vi "Quality_Traceability.vi"() -> ()   [LabVIEW 2020]
doc: "Fonction :\n\nCe modèle peut être intégré très facilement à un subpannel à l'aide des fonctions de la palette Code Template >> Dynamic VI and Subpanel de la VIBOX"
uses:
  System.Windows.Forms
  <vilib>/Utility/NIReport.llb/Report Type.ctl
  <vilib>/Utility/NIReport.llb/Append Text Table to Report (wrap).vi
  <vilib>/DataGrid for LabVIEW/source/DataTable/DataTable.lvclass
  <vilib>/DataGrid for LabVIEW/source/DataGridView/DataGridView.lvclass
  C:/Program Files (x86)/National Instruments/LabVIEW 2020/examples/DataGrid for LabVIEW/DataGrid.lvlib
  <vilib>/DataGrid for LabVIEW/source/Events/CellClick/CellClick.lvclass
  <vilib>/Utility/NIReport.llb/NI_report.lvclass
  <vilib>/Utility/NIReport.llb/NI_ReportGenerationCore.lvlib
panel:
  out "data":string[][](array[string])
  in  "截至日期":timestamp format="%<%x>T"
  in  "起始日期":timestamp caption="日期范围" format="%<%x>T"
  out "Stop":bool
  out "row":i32
  in  "加工状态":u16(ring) caption="Enum 3" items=["", "OK", "NG"]
  in  "生产编号":string
  in  "操作员":string
  in  "产品型号":u16(ring) caption="Enum 3" items=["", "R128", "R527", "R538", "R544", "R563X", "R92A"]
  in  "设备名称":u16(ring) caption="Enum 3" items=["", "芯轴分总成磨合台", "上管柱组件装配", "上管柱上转向轴合成", "滑移力检测", "芯轴分总成NVH", "上转向轴组件装配", "上下管柱总成装配", "滑移力复检", "最终性能试验台", "传感器对中台", "电机装配", "中间轴装配", "GP12（340）", "ECU装配", "激光打标机"]
  in  "追溯码":string
  in  "详细信息":bool
  in  "搜索按钮":bool
  out "Stop<user event>":refnum<user-event>
  in  "质量追溯":refnum<k24>(container)
  in  "导出全部行":bool
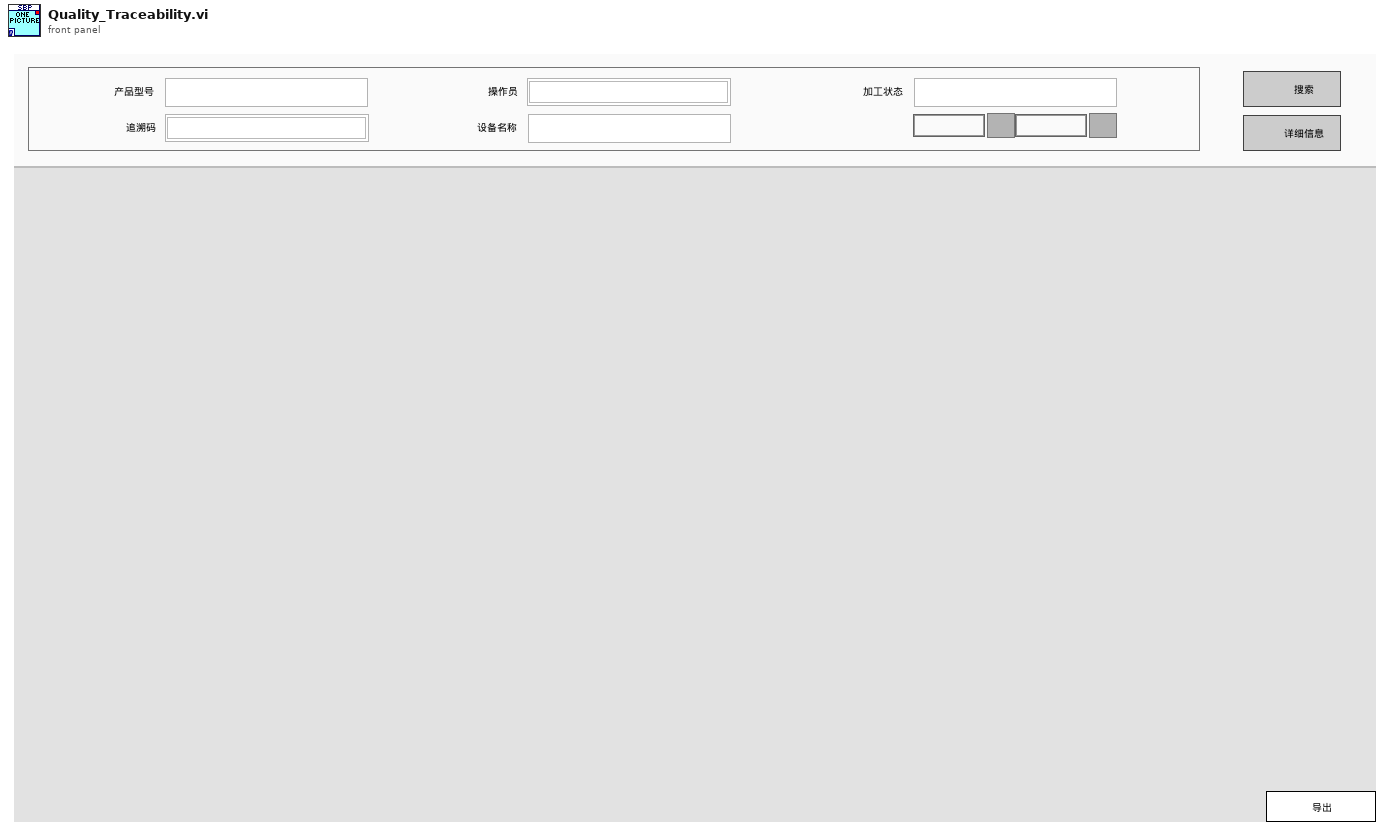
[diagram p1: front panel]
types:
  T1 = typedef "NI_ReportGenerationCore.lvlib/Report Type.ctl" = enum16{"HTML", "Word", "Excel"}
  T2 = enum16{"maximized", "minimized", "normal", "no change"}
  T3 = typedef "DataGrid.lvlib/GridColumn.lvclass/ColumnDefinition.ctl" = cluster{"name":string, "caption":string, "datatype":T4, "Params":string, "AutoSizeMode":i32, "FillWeight":sgl, "MinWidth":u32, "tooltip":string}
  T4 = typedef "DataGrid.lvlib/GridColumn.lvclass/ColumnType.ctl" = enum16{"string", "image", "check", "numeric", "timestamp", "button", "combo", "link"}
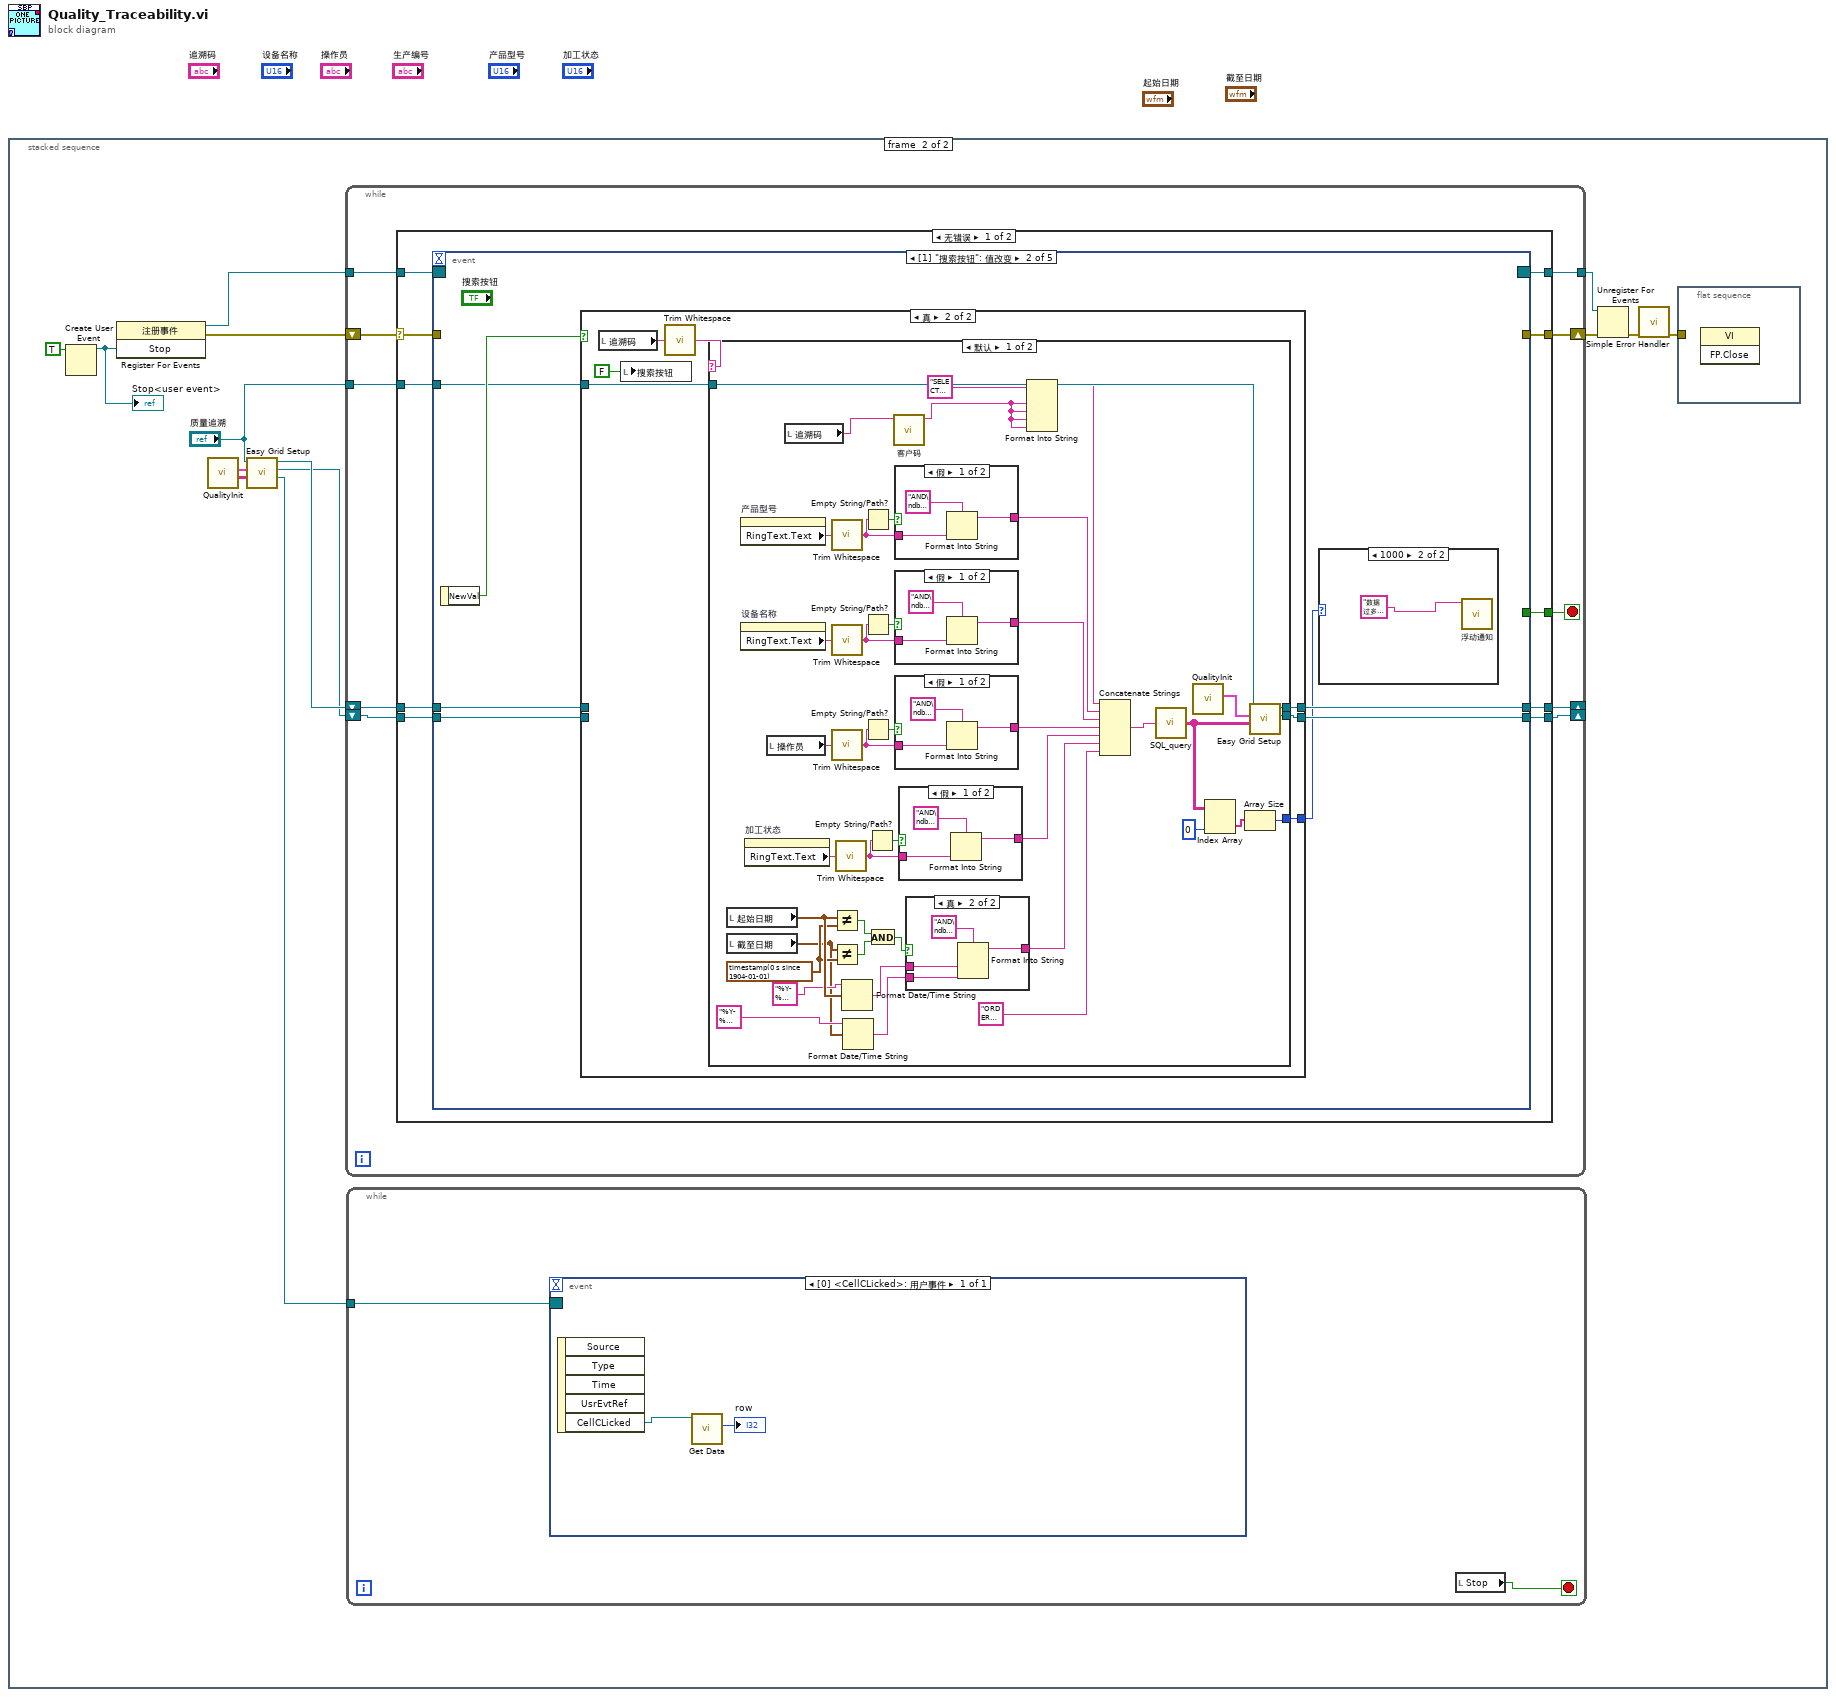
[diagram p0: block diagram]
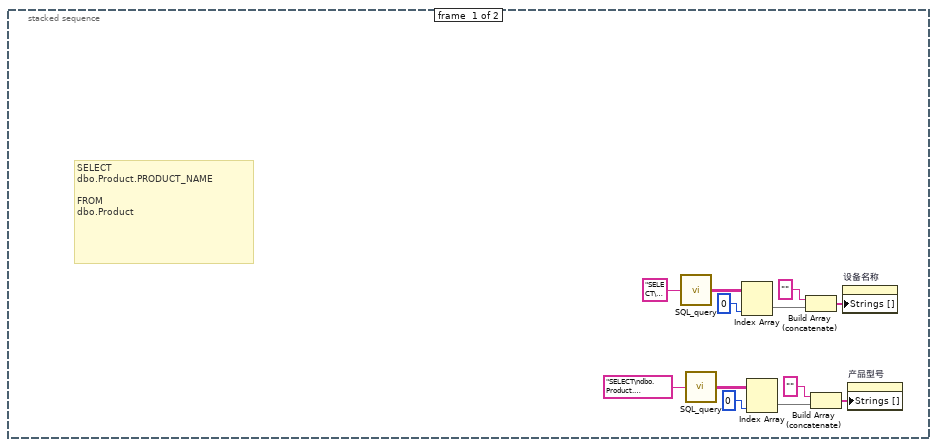
[diagram p2: hidden frame]
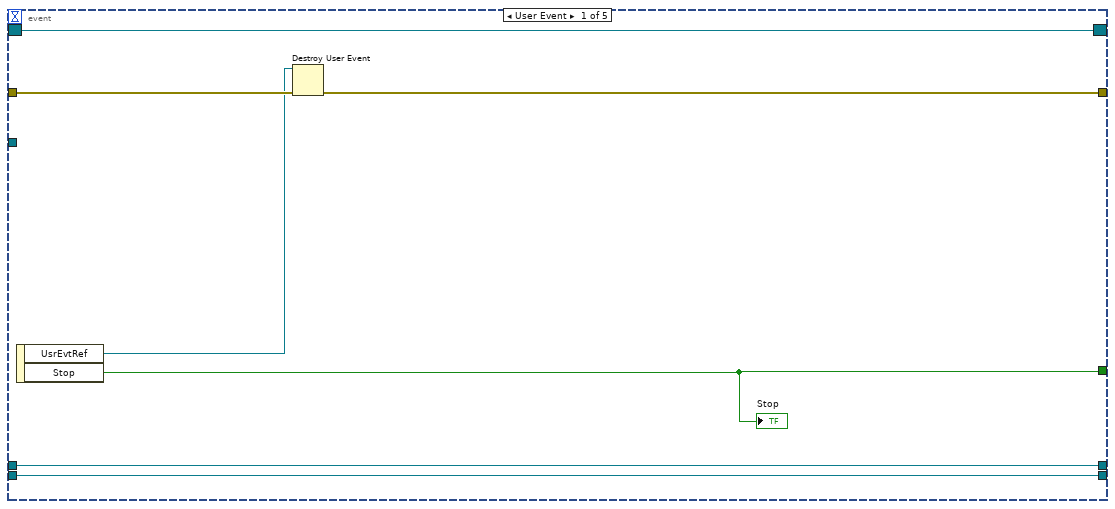
[diagram p3: hidden frame]
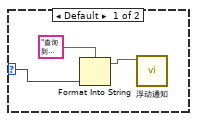
[diagram p4: hidden frame]
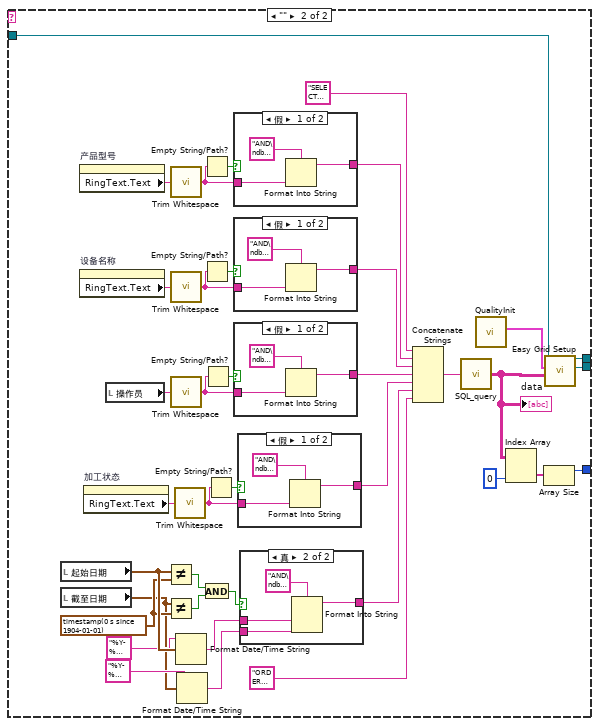
[diagram p11: hidden frame]
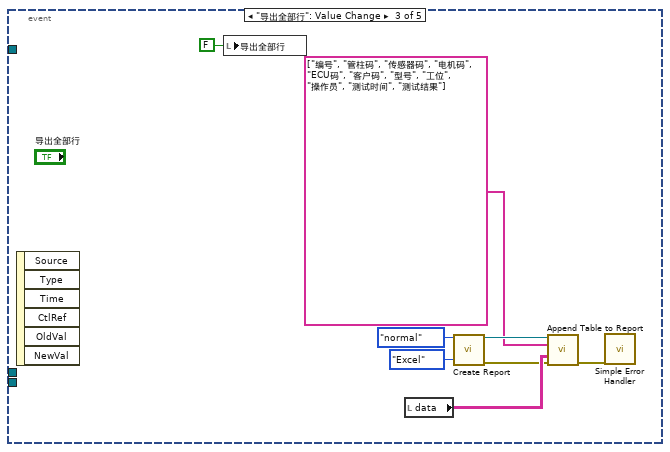
[diagram p17: hidden frame]
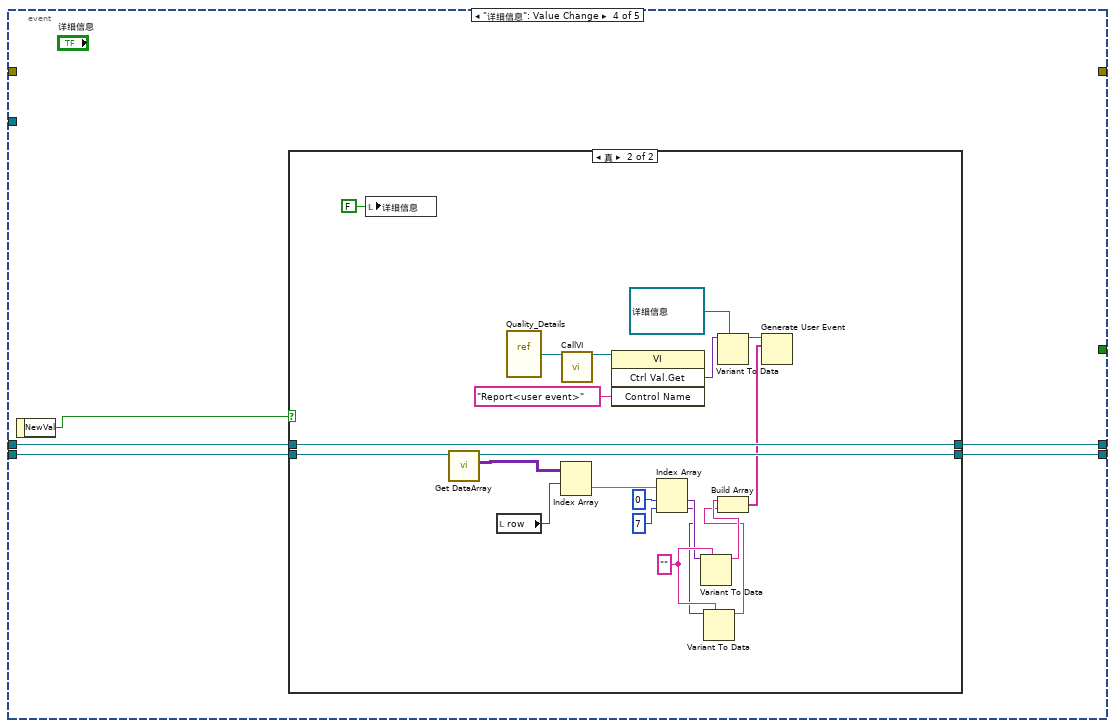
[diagram p18: hidden frame]
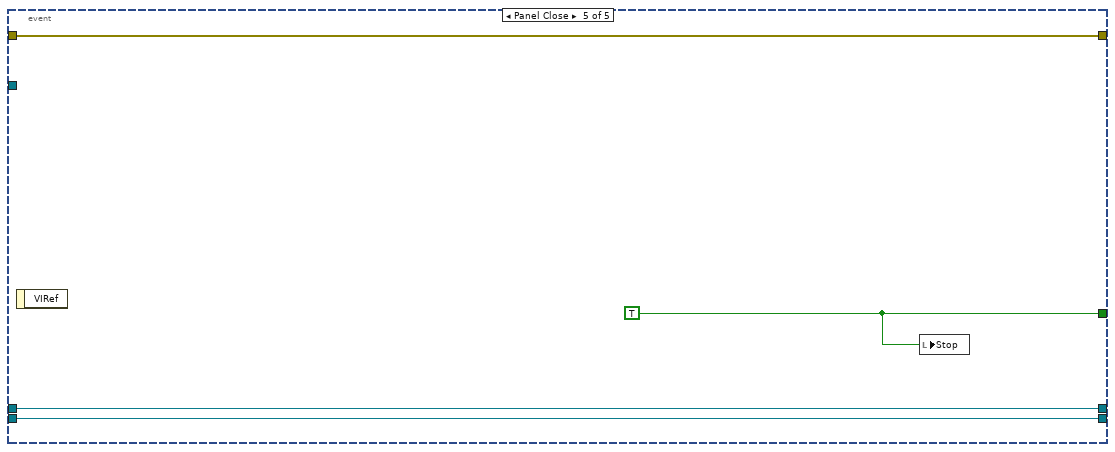
[diagram p20: hidden frame]
diagram:
  n1 = stacked-sequence {
    frame #0 {
      # "SELECT\ndbo.Product.PRODUCT_NAME\n\nFROM\ndbo.Product"
      n2 = call "SQL_query.vi"("SQL query"="SELECT\ndbo.Device.DEVICE_NAME\n\nFROM\ndbo.Device\n") -> ("data"=w11:string[][])  [unwired: 3 in, 1 out]
      n3 = call "SQL_query.vi"("SQL query"="SELECT\ndbo.Product.PRODUCT_NAME\n\nFROM\ndbo.Product\n") -> ("data"=w3:string[][])  [unwired: 3 in, 1 out]
      n4 = Index Array(array=w11, index (col)=0 ("禁用的索引 (列)")) -> (element=w10:string[])  [unwired: 1 in]
      n5 = Index Array(array=w3, index (col)=0 ("禁用的索引 (列)")) -> (element=w4:string[])  [unwired: 1 in]
      n6 = Build Array (concatenate)("", w10) -> (w8:string[])
      n7 = Build Array (concatenate)("", w4) -> (w1:string[])
      n8 = property on="设备名称" class="Ring (严格)"("Strings []"=w8) -> ()  [unwired: 2 in, 2 out]
      n9 = property on="产品型号" class="Ring (严格)"("Strings []"=w1) -> ()  [unwired: 2 in, 2 out]
    }
    frame #1 {
      n10 = Create User Event(user event datatype=TRUE ("Stop")) -> (user event=w24:refnum<user-event>)  [unwired: 1 in, 1 out]
      "Stop<user event>" <- w24
      n11 = register-events(w24) -> (reference out=w23:refnum<event-registration>, error out=w19:errorcluster)  [unwired: 2 in]
      n12 = call "QualityInit.vi"() -> ("DataSource Data"=w17:string[][], "ColumnSetup"=w18:T3[])  [unwired: 10 in]
      n13 = call <vilib>:"Easy Grid Setup.vi"("DataSource Data"=w17, "ColumnSetup"=w18, "DataGridView"="质量追溯") -> ("registeredEvents"=w15:refnum<event-registration>, "DataTable out"=w13:refnum<class "DataTable.lvclass">, "DataGrid out"=w14:refnum<class "DataGridView.lvclass">)  [unwired: 5 in, 1 out]
      n14 = while {
        tunnel: w23 -> [w37]
        tunnel: [w36] -> w26
        shift-right: [w39] -> w22
        shift-left: w19 -> [w40]
        tunnel: "质量追溯" -> [w35]
        shift-right: [w34] -> _
        shift-left: w14 -> [w32]
        shift-right: [w33] -> _
        shift-left: w13 -> [w31]
        stop <- w38 stop-if-true
        n15 = case shown="无错误" w40 {
          selector: w40 -> [w47 w232]
          tunnel: [w46 w232] -> w39
          tunnel: [w48 TRUE] -> w38
          tunnel: w37 -> [w49 w231]
          tunnel: [w50 w231] -> w36
          tunnel: w35 -> [w45 _]
          tunnel: [w44 w230] -> w34
          tunnel: [w43 w229] -> w33
          tunnel: w32 -> [w42 w230]
          tunnel: w31 -> [w41 w229]
          frame No Error {
            n16 = event shown="[1] \"搜索按钮\": 值改变" {
              selector: w49 -> [w57 _ _ _ _]
              dyn-events: [w57 _ _ _ _] -> w50
              timeout: _ -> [_ _ _ _ _]
              tunnel: [w54 _ _ _ w227] -> w48
              tunnel: w47 -> [w56 _ _ _ w228]
              tunnel: [w53 _ _ _ w228] -> w46
              tunnel: w45 -> [_ w63 _ _ _]
              tunnel: [w52 w62 _ w199 w226] -> w44
              tunnel: [w51 w61 _ w197 w225] -> w43
              tunnel: w42 -> [w52 w60 _ w200 w226]
              tunnel: w41 -> [w51 w59 _ w198 w225]
              event User Event {
                n17 = event-data() -> ("UsrEvtRef"=w55:refnum<user-event>, "Stop"=w54:bool)  [unwired: 1 out]
                "Stop" <- w54
                n18 = Destroy User Event(user event=w55, error in=w56) -> (error out=w53:errorcluster)
              }
              event "搜索按钮": Value Change {
                n19 = event-data() -> ("NewVal"=w64:bool)  [unwired: 1 out]
                n20 = case shown="真" w64 {
                  tunnel: w63 -> [_ w76]
                  tunnel: [w70 w73] -> w62
                  tunnel: [w69 w72] -> w61
                  tunnel: w60 -> [w70 _]
                  tunnel: w59 -> [w69 _]
                  tunnel: [_ w71] -> w58
                  frame False {
                  }
                  frame True {
                    n21 = local read "追溯码"() -> (w75:string)
                    n22 = local write "搜索按钮"(FALSE ("确定按钮")) -> ()
                    n23 = call <vilib>:"Trim Whitespace.vi"("string"=w75) -> ("trimmed string"=w74:string)  [unwired: 1 in]
                    n24 = case shown="默认" w74 {
                      tunnel: w76 -> [w108 w172]
                      tunnel: [w99 w170] -> w73
                      tunnel: [w98 w169] -> w72
                      tunnel: [w81 w136] -> w71
                      frame Default {
                        w87 = timestamp(0 s since 1904-01-01) ("起始日期")
                        n25 = local read "起始日期"() -> (w90:timestamp)
                        n26 = local read "截至日期"() -> (w82:timestamp)
                        n27 = property on="产品型号" class="Ring (严格)"() -> ("RingText.Text"=w118:string)  [unwired: 2 in, 2 out]
                        n28 = property on="设备名称" class="Ring (严格)"() -> ("RingText.Text"=w117:string)  [unwired: 2 in, 2 out]
                        n29 = property on="加工状态" class="Ring (严格)"() -> ("RingText.Text"=w102:string)  [unwired: 2 in, 2 out]
                        n30 = local read "操作员"() -> (w116:string)
                        n31 = local read "追溯码"() -> (w96:string)
                        n32 = call <vilib>:"Trim Whitespace.vi"("string"=w118) -> ("trimmed string"=w106:string)  [unwired: 1 in]
                        n33 = call <vilib>:"Trim Whitespace.vi"("string"=w117) -> ("trimmed string"=w105:string)  [unwired: 1 in]
                        n34 = call <vilib>:"Trim Whitespace.vi"("string"=w116) -> ("trimmed string"=w104:string)  [unwired: 1 in]
                        n35 = Not Equal?(x=w90, y=w87) -> (x != y?=w92:bool)
                        n36 = Not Equal?(x=w82, y=w87) -> (x != y?=w93:bool)
                        n37 = call <vilib>:"Trim Whitespace.vi"("string"=w102) -> ("trimmed string"=w101:string)  [unwired: 1 in]
                        n38 = Format Date/Time String(time format string (%c)="%Y-%m-%d 00:00:00.000" ("时间格式字符串(%c)"), seconds (now)=w90) -> (date/time string=w89:string)  [unwired: 1 in]
                        n39 = Format Date/Time String(time format string (%c)="%Y-%m-%d 23:59:59.999" ("时间格式字符串(%c)"), seconds (now)=w82) -> (date/time string=w88:string)  [unwired: 1 in]
                        n40 = Empty String/Path?(string/path=w106) -> (empty?=w113:bool)
                        n41 = Empty String/Path?(string/path=w105) -> (empty?=w114:bool)
                        n42 = Empty String/Path?(string/path=w104) -> (empty?=w115:bool)
                        n43 = Empty String/Path?(string/path=w101) -> (empty?=w103:bool)
                        n44 = And(x=w92, y=w93) -> (x .and. y?=w91:bool)
                        n45 = call "客户码.vi"("追溯码"=w96) -> ("追溯码 2"=w95:string)  [unwired: 10 in]
                        n46 = case shown="假" w113 {
                          tunnel: [w133 _] -> w112
                          tunnel: w106 -> [w134 _]
                          frame False {
                            n47 = Format Into String(format string="AND\ndbo.Product.PRODUCT_NAME = '%s'\n" ("输入 1"), w134) -> (resulting string=w133:string)  [unwired: 2 in, 1 out]
                          }
                          frame True {
                          }
                        }
                        n48 = case shown="假" w114 {
                          tunnel: [w130 _] -> w111
                          tunnel: w105 -> [w131 _]
                          frame False {
                            n49 = Format Into String(format string="AND\ndbo.Device.DEVICE_NAME = '%s'" ("输入 1"), w131) -> (resulting string=w130:string)  [unwired: 2 in, 1 out]
                          }
                          frame True {
                          }
                        }
                        n50 = case shown="假" w115 {
                          tunnel: [w127 _] -> w110
                          tunnel: w104 -> [w128 _]
                          frame False {
                            n51 = Format Into String(format string="AND\ndbo.[User].USER_NAME = '%s'\n" ("输入 1"), w128) -> (resulting string=w127:string)  [unwired: 2 in, 1 out]
                          }
                          frame True {
                          }
                        }
                        n52 = case shown="假" w103 {
                          tunnel: [w124 _] -> w100
                          tunnel: w101 -> [w125 _]
                          frame False {
                            n53 = Format Into String(format string="AND\ndbo.Result.RESULT_VALUE = '%s'" ("输入 1"), w125) -> (resulting string=w124:string)  [unwired: 2 in, 1 out]
                          }
                          frame True {
                          }
                        }
                        n54 = case shown="真" w91 {
                          tunnel: [_ w121] -> w84
                          tunnel: w89 -> [_ w122]
                          tunnel: w88 -> [_ w119]
                          frame False {
                          }
                          frame True {
                            n55 = Format Into String(format string="AND\ndbo.Result.RESULT_TIME BETWEEN '%s' AND '%s'" ("输入 1"), w122, w119) -> (resulting string=w121:string)  [unwired: 2 in, 1 out]
                          }
                        }
                        n56 = Format Into String(format string="SELECT top 1000 \ndbo.Code.CODE_ID,\ndbo.Code.CODE_MAIN,\ndbo.Code.CODE_SENSOR,\ndbo.Code.CODE_MOTOR,\ndbo.Code.CODE_ECU,\ndbo.Code_Custom.CODE_CUSTOM,\ndbo.Product.PRODUCT_NAME,\ndbo.Device.DEVICE_NAME,\ndbo.[User].USER_NAME,\ndbo.Result.RESULT_TIME,\ndbo.Result.RESULT_VALUE\n\nFROM\ndbo.Result\nINNER JOIN dbo.Code ON dbo.Result.CODE_ID = dbo.Code.CODE_ID\nINNER JOIN dbo.[User] ON dbo.Result.USER_ID = dbo.[User].USER_ID\nINNER JOIN dbo.Product ON dbo.Code.PRODUCT_ID = dbo.Product.PRODUCT_ID\nINNER JOIN dbo.Device ON dbo.Result.DEVICE_ID = dbo.Device.DEVICE_ID\nLEFT JOIN dbo.Code_Custom ON dbo.Code_Custom.CODE_MAIN = dbo.Code.CODE_MAIN\nWHERE\n(dbo.Code.CODE_MAIN LIKE '%%%s%%' OR\ndbo.Code.CODE_SENSOR LIKE '%%%s%%' OR\ndbo.Code.CODE_MOTOR LIKE '%%%s%%' OR\ndbo.Code.CODE_ECU LIKE '%%%s%%'\n)" ("字符串"), w95, w95, w95, w95) -> (resulting string=w97:string)  [unwired: 2 in, 1 out]
                        n57 = Concatenate Strings(w97, w112, w111, w110, w100, w84, "ORDER BY\ndbo.Code.CODE_ID DESC" ("字符串")) -> (w109:string)
                        n58 = call "SQL_query.vi"("SQL query"=w109) -> ("data"=w80:string[][])  [unwired: 3 in, 1 out]
                        n59 = call "QualityInit.vi"() -> ("ColumnSetup"=w107:T3[])  [unwired: 10 in, 1 out]
                        n60 = Index Array(array=w80, index (col)=0 ("禁用的索引 (列)")) -> (element=w78:string[])  [unwired: 1 in]
                        n61 = Array Size(array=w78) -> (size(s)=w81:i32)
                        n62 = call <vilib>:"Easy Grid Setup.vi"("DataSource Data"=w80, "ColumnSetup"=w107, "DataGridView"=w108) -> ("DataTable out"=w98:refnum<class "DataTable.lvclass">, "DataGrid out"=w99:refnum<class "DataGridView.lvclass">)  [unwired: 5 in, 2 out]
                      }
                      frame "" {
                        w144 = timestamp(0 s since 1904-01-01) ("起始日期")
                        n63 = local read "起始日期"() -> (w147:timestamp)
                        n64 = local read "截至日期"() -> (w139:timestamp)
                        n65 = property on="产品型号" class="Ring (严格)"() -> ("RingText.Text"=w168:string)  [unwired: 2 in, 2 out]
                        n66 = property on="设备名称" class="Ring (严格)"() -> ("RingText.Text"=w167:string)  [unwired: 2 in, 2 out]
                        n67 = property on="加工状态" class="Ring (严格)"() -> ("RingText.Text"=w155:string)  [unwired: 2 in, 2 out]
                        n68 = local read "操作员"() -> (w166:string)
                        n69 = Not Equal?(x=w147, y=w144) -> (x != y?=w149:bool)
                        n70 = Not Equal?(x=w139, y=w144) -> (x != y?=w150:bool)
                        n71 = call <vilib>:"Trim Whitespace.vi"("string"=w168) -> ("trimmed string"=w159:string)  [unwired: 1 in]
                        n72 = call <vilib>:"Trim Whitespace.vi"("string"=w167) -> ("trimmed string"=w158:string)  [unwired: 1 in]
                        n73 = call <vilib>:"Trim Whitespace.vi"("string"=w166) -> ("trimmed string"=w157:string)  [unwired: 1 in]
                        n74 = call <vilib>:"Trim Whitespace.vi"("string"=w155) -> ("trimmed string"=w154:string)  [unwired: 1 in]
                        n75 = Format Date/Time String(time format string (%c)="%Y-%m-%d 00:00:00.000" ("时间格式字符串(%c)"), seconds (now)=w147) -> (date/time string=w143:string)  [unwired: 1 in]
                        n76 = Format Date/Time String(time format string (%c)="%Y-%m-%d 23:59:59.999" ("时间格式字符串(%c)"), seconds (now)=w139) -> (date/time string=w142:string)  [unwired: 1 in]
                        n77 = Empty String/Path?(string/path=w159) -> (empty?=w163:bool)
                        n78 = Empty String/Path?(string/path=w158) -> (empty?=w164:bool)
                        n79 = And(x=w149, y=w150) -> (x .and. y?=w148:bool)
                        n80 = Empty String/Path?(string/path=w157) -> (empty?=w165:bool)
                        n81 = Empty String/Path?(string/path=w154) -> (empty?=w156:bool)
                        n82 = case shown="假" w163 {
                          tunnel: [w187 _] -> w162
                          tunnel: w159 -> [w188 _]
                          frame False {
                            n83 = Format Into String(format string="AND\ndbo.Product.PRODUCT_NAME = '%s'\n" ("输入 1"), w188) -> (resulting string=w187:string)  [unwired: 2 in, 1 out]
                          }
                          frame True {
                          }
                        }
                        n84 = case shown="假" w164 {
                          tunnel: [w184 _] -> w161
                          tunnel: w158 -> [w185 _]
                          frame False {
                            n85 = Format Into String(format string="AND\ndbo.Device.DEVICE_NAME = '%s'" ("输入 1"), w185) -> (resulting string=w184:string)  [unwired: 2 in, 1 out]
                          }
                          frame True {
                          }
                        }
                        n86 = case shown="假" w165 {
                          tunnel: [w181 _] -> w160
                          tunnel: w157 -> [w182 _]
                          frame False {
                            n87 = Format Into String(format string="AND\ndbo.[User].USER_NAME = '%s'\n" ("输入 1"), w182) -> (resulting string=w181:string)  [unwired: 2 in, 1 out]
                          }
                          frame True {
                          }
                        }
                        n88 = case shown="假" w156 {
                          tunnel: [w178 _] -> w153
                          tunnel: w154 -> [w179 _]
                          frame False {
                            n89 = Format Into String(format string="AND\ndbo.Result.RESULT_VALUE = '%s'" ("输入 1"), w179) -> (resulting string=w178:string)  [unwired: 2 in, 1 out]
                          }
                          frame True {
                          }
                        }
                        n90 = case shown="真" w148 {
                          tunnel: [_ w175] -> w141
                          tunnel: w143 -> [_ w176]
                          tunnel: w142 -> [_ w173]
                          frame False {
                          }
                          frame True {
                            n91 = Format Into String(format string="AND\ndbo.Result.RESULT_TIME BETWEEN '%s' AND '%s'" ("输入 1"), w176, w173) -> (resulting string=w175:string)  [unwired: 2 in, 1 out]
                          }
                        }
                        n92 = Concatenate Strings("SELECT top 1000 \ndbo.Code.CODE_ID,\ndbo.Code.CODE_MAIN,\ndbo.Code.CODE_SENSOR,\ndbo.Code.CODE_MOTOR,\ndbo.Code.CODE_ECU,\ndbo.Code_Custom.CODE_CUSTOM,\ndbo.Product.PRODUCT_NAME,\ndbo.Device.DEVICE_NAME,\ndbo.[User].USER_NAME,\ndbo.Result.RESULT_TIME,\ndbo.Result.RESULT_VALUE\n\nFROM\ndbo.Result\nINNER JOIN dbo.Code ON dbo.Result.CODE_ID = dbo.Code.CODE_ID\nINNER JOIN dbo.[User] ON dbo.Result.USER_ID = dbo.[User].USER_ID\nINNER JOIN dbo.Product ON dbo.Code.PRODUCT_ID = dbo.Product.PRODUCT_ID\nINNER JOIN dbo.Device ON dbo.Result.DEVICE_ID = dbo.Device.DEVICE_ID\nLEFT JOIN dbo.Code_Custom ON dbo.Code_Custom.CODE_MAIN = dbo.Code.CODE_MAIN\nWHERE\n1=1\n" ("字符串"), w162, w161, w160, w153, w141, "ORDER BY\ndbo.Code.CODE_ID DESC" ("字符串")) -> (w152:string)
                        n93 = call "SQL_query.vi"("SQL query"=w152) -> ("data"=w135:string[][])  [unwired: 3 in, 1 out]
                        "data" <- w135
                        n94 = call "QualityInit.vi"() -> ("ColumnSetup"=w171:T3[])  [unwired: 10 in, 1 out]
                        n95 = Index Array(array=w135, index (col)=0 ("禁用的索引 (列)")) -> (element=w138:string[])  [unwired: 1 in]
                        n96 = Array Size(array=w138) -> (size(s)=w136:i32)
                        n97 = call <vilib>:"Easy Grid Setup.vi"("DataSource Data"=w135, "ColumnSetup"=w171, "DataGridView"=w172) -> ("DataTable out"=w169:refnum<class "DataTable.lvclass">, "DataGrid out"=w170:refnum<class "DataGridView.lvclass">)  [unwired: 5 in, 2 out]
                      }
                    }
                  }
                }
                n98 = case shown="1000" w58 {
                  selector: w58 -> [w65 _]
                  frame Default {
                    n99 = Format Into String(format string="查询到%d条记录", w65) -> (resulting string=w67:string)  [unwired: 2 in, 1 out]
                    n100 = call "浮动通知.vi"("通知内容"=w67) -> ()  [unwired: 11 in]
                  }
                  frame 1000 {
                    n101 = call "浮动通知.vi"("通知内容"="数据过多，仅显示最近1000条记录！") -> ()  [unwired: 11 in]
                  }
                }
              }
              event "导出全部行": Value Change {
                n102 = event-data() -> ()  [unwired: 7 out]
                n103 = local write "导出全部行"(FALSE ("导出全部行")) -> ()
                n104 = local read "data"() -> (w192:string[][])
                n105 = call <vilib>:"Create Report.vi"("window state (normal)"=T2."normal", "report type"=Report_Type."Excel") -> ("report out"=w193:refnum<class "NI_report.lvclass">, "error out"=w191:errorcluster)  [unwired: 12 in]
                n106 = call-poly <vilib>:"Append Table to Report.vi"("report in"=w193, "column headers"=string[] ["编号", "管柱码", "传感器码", "电机码", "ECU码", "客户码", "型号", "工位", "操作员", "测试时间", "测试结果"] ("row headers"), "text data"=w192, "error in (no error)"=w191) -> ("error out"=w189:errorcluster)  [unwired: 8 in, 3 out]
                n107 = call <vilib>:"Simple Error Handler.vi"("error in (no error)"=w189) -> ()  [unwired: 4 in, 5 out]
              }
              event "详细信息": Value Change {
                n108 = event-data() -> ("NewVal"=w201:bool)  [unwired: 1 out]
                n109 = case shown="真" w201 {
                  tunnel: w200 -> [w203 w217]
                  tunnel: [w203 w217] -> w199
                  tunnel: w198 -> [w202 w216]
                  tunnel: [w202 w215] -> w197
                  frame False {
                  }
                  frame True {
                    w208 = ""
                    n110 = local write "详细信息"(FALSE ("更多按钮")) -> ()
                    n111 = call <vilib>:"Get DataArray.vi"("DataTable in"=w216) -> ("Array"=w209:variant[][], "DataTable out"=w215:refnum<class "DataTable.lvclass">)  [unwired: 8 in, 1 out]
                    n112 = local read "row"() -> (w214:i32)
                    n113 = vi-ref "Quality_Details.vi"() -> (w219:refnum<vi>)
                    n114 = Index Array(array=w209, index (row)=w214) -> (element=w213:variant[])  [unwired: 1 in]
                    n115 = call "CallVI.vi"("VI引用"=w219) -> ("VI引用输出"=w218:refnum<vi>)  [unwired: 12 in, 2 out]
                    n116 = invoke class="VI" method="Ctrl Val.Get"(reference=w218, "Control Name"="Report<user event>" ("控件名")) -> ("Get Control Value Variant"=w222:variant)  [unwired: 2 in, 3 out]
                    n117 = Index Array(array=w213, index #1=0 ("索引"), index #2=7 ("索引")) -> (element #1=w207:variant, element #2=w205:variant)
                    n118 = Variant To Data(type=w208, Variant=w207) -> (data=w206:string)  [unwired: 1 in, 1 out]
                    n119 = Variant To Data(type=w208, Variant=w205) -> (data=w204:string)  [unwired: 1 in, 1 out]
                    n120 = Variant To Data(type=refnum<user-event> refnum ("Report<user event>"), Variant=w222) -> (data=w220:refnum<user-event>)  [unwired: 1 in, 1 out]
                    n121 = Build Array(w206, w204) -> (w210:string[])
                    n122 = Generate User Event(user event=w220, event data cluster=w210) -> ()  [unwired: 2 in, 2 out]
                  }
                }
              }
              event Panel Close {
                w227 = TRUE ("Stop")
                n123 = event-data() -> ()  [unwired: 2 out]
                n124 = local write "Stop"(w227) -> ()
              }
            }
          }
          frame Error {
          }
        }
      }
      n125 = while {
        tunnel: w15 -> [w28]
        stop <- w27 stop-if-true
        n126 = event shown="[0] <CellCLicked>: 用户事件" {
          selector: w28 -> [_]
          dyn-events: _ -> [_]
          timeout: _ -> [_]
          event User Event {
            n127 = event-data() -> ("CellCLicked"=w30:refnum<class "Abstract EVENT.lvclass">)  [unwired: 1 in, 4 out]
            n128 = call <vilib>:"Get Data.vi"("DataGrid.lvlib:Abstract EVENT.lvclass"=w30) -> ("row"=→"row":i32)  [unwired: 8 in, 2 out]
          }
        }
        n129 = local read "Stop"() -> (w27:bool)
      }
      n130 = Unregister For Events(event registration refnum=w26, error in=w22) -> (error out=w25:errorcluster)
      n131 = call <vilib>:"Simple Error Handler.vi"("error in (no error)"=w25) -> ("error out"=w20:errorcluster)  [unwired: 1 in, 7 out]
      n132 = flat-sequence {
        tunnel: w20 -> [_]
        frame #0 {
          n133 = invoke class="VI" method="FP.Close"() -> ()  [unwired: 3 in, 3 out]
        }
      }
    }
  }
